vi "Debug JSON Response.vi"(8 "error in (no error)":errorcluster, 9 "timeout in ms (1000)":i32=1000, 10 "Client Message":refnum<class "Client Message.lvclass">, 11 "OBS in":refnum<class "OBS.lvclass">) -> (0 "error out":errorcluster, 1 "Has Response?":bool, 2 "JSON Response":string, 3 "OBS out":refnum<class "OBS.lvclass">)   [LabVIEW 2020, in "obs-websocket.lvlib" / "OBS.lvclass"]
uses:
  OBS.lvclass
  OBS.lvclass/OBS.ctl
  RJSONDebug/RJSONDebug.lvclass
  C:/dev/lv20CE/relink/lv-obs-websocket/obs-websocket/Response/Response.lvclass
  C:/dev/lv20CE/relink/lv-obs-websocket/obs-websocket/Server Message/Server Message.lvclass
  C:/dev/lv20CE/relink/lv-obs-websocket/obs-websocket/Message/Message.lvclass
  C:/dev/lv20CE/relink/lv-promises/Promises/Value/Value.lvclass
  C:/dev/lv20CE/relink/lv-obs-websocket/obs-websocket/RJSONDebug/RJSONDebug.lvclass
  Client Message/Client Message.lvclass
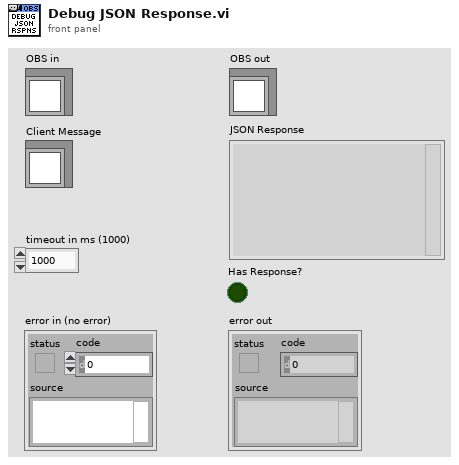
[diagram p1: front panel]
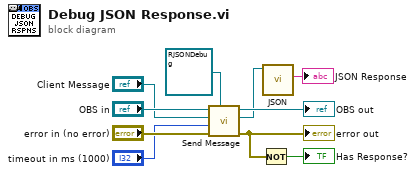
[diagram p0: block diagram]
diagram:
  n1 = call "Send Message.vi"("Response Type (None)"=refnum<class "RJSONDebug.lvclass"> refnum ("obs-websocket.lvlib:RJSONDebug.lvclass"), "error in (no error)"="error in (no error)", "timeout in ms (1000)"="timeout in ms (1000)", "Client Message"="Client Message", "OBS in"="OBS in") -> ("error out"=w4:errorcluster, "Response"=w6:refnum<class "RJSONDebug.lvclass">, "OBS out"=→"OBS out":refnum<class "OBS.lvclass">)  [unwired: 3 in, 1 out]
  "error out" <- w4
  n2 = Not(x=w4) -> (.not. x?=→"Has Response?":bool)
  n3 = call "JSON.vi"("RJSONDebug in"=w6) -> ("JSON"=→"JSON Response":string)  [unwired: 8 in, 2 out]
